vi "Get Service Class Instances.vi"() -> (3 "service instances":refnum<class "ServiceBase.lvclass">[](array[class]))   [LabVIEW 2019, in "MicronGRPCGeneratedServer.lvlib"]
uses:
  MicronGRPCGeneratedServer.lvlib
  <vilib>/gRPC/LabVIEW gRPC Servicer/ServiceBase/ServiceBase.lvclass
  RPC Service/MicronGRPC/MicronGRPC.lvclass
  C:/Program Files (x86)/National Instruments/LabVIEW 2019/vi.lib/gRPC/LabVIEW gRPC Servicer/ServiceBase/ServiceBase.lvclass
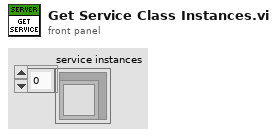
[diagram p1: front panel]
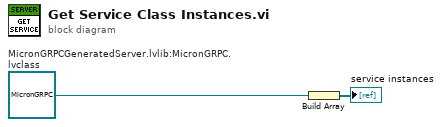
[diagram p0: block diagram]
diagram:
  w1 = refnum<class "MicronGRPC.lvclass"> refnum  # MicronGRPCGeneratedServer.lvlib:MicronGRPC.lvclass
  n1 = Build Array(w1) -> (→"service instances":refnum<class "MicronGRPC.lvclass">[])
